vi "EminemNetworking.vi"(8 "error in (no error)":errorcluster) -> (0 "error out":errorcluster)   [LabVIEW 2023]
uses:
  EminemGlobals.vi
  <vilib>/Rock Robotics/Network Tables/NT Write Boolean.vi
  <vilib>/Rock Robotics/Network Tables/NT Write Number.vi
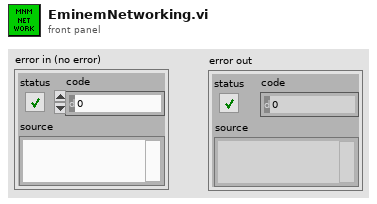
[diagram p1: front panel]
types:
  T1 = typedef "EminemStatesEnum.ctl" = enum16{"0-Init", "1-WaitForCmd", "2-Cancel", "3-ShootStart", "4-ShootRev", "5-RevUpStart", "6-ShootStartFeed&Timer", "7-ShootTimerOrSensorDone", "8-ShootDone", "9-AmpStart", "10-AmpUpToSpd?", "11-AmpStartFeed&Timer", "12-AmpTimerOrSensorDone", "13-AmpDone", "14-RevUpGetCmd"}
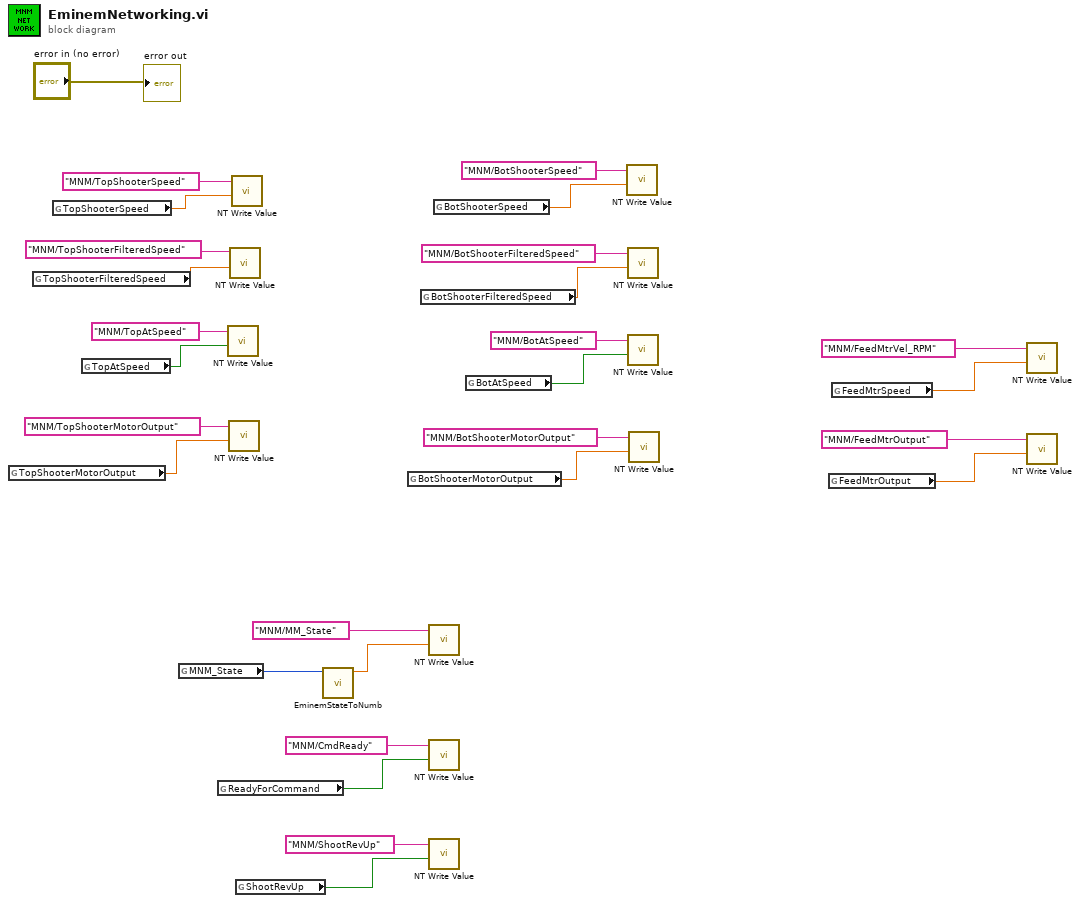
[diagram p0: block diagram]
diagram:
  n1 = global read "EminemGlobals.vi" "TopShooterMotorOutput"() -> (w12:dbl)
  n2 = global read "EminemGlobals.vi" "TopShooterFilteredSpeed"() -> (w18:dbl)
  n3 = global read "EminemGlobals.vi" "TopShooterSpeed"() -> (w17:dbl)
  n4 = global read "EminemGlobals.vi" "TopAtSpeed"() -> (w16:bool)
  n5 = global read "EminemGlobals.vi" "MNM_State"() -> (w7:T1)
  n6 = global read "EminemGlobals.vi" "ReadyForCommand"() -> (w10:bool)
  n7 = call-poly <vilib>:"NT Write Value.vi"("value"=w16, "name"="MNM/TopAtSpeed") -> ()  [unwired: 9 in, 1 out]
  n8 = call-poly <vilib>:"NT Write Value.vi"("value"=w12, "name"="MNM/TopShooterMotorOutput") -> ()  [unwired: 9 in, 1 out]
  n9 = call-poly <vilib>:"NT Write Value.vi"("value"=w18, "name"="MNM/TopShooterFilteredSpeed") -> ()  [unwired: 9 in, 1 out]
  n10 = call-poly <vilib>:"NT Write Value.vi"("value"=w17, "name"="MNM/TopShooterSpeed") -> ()  [unwired: 9 in, 1 out]
  n11 = global read "EminemGlobals.vi" "ShootRevUp"() -> (w1:bool)
  n12 = call "EminemStateToNumb.vi"("Eminim_state"=w7) -> ("StateNumber"=w5:dbl)  [unwired: 10 in]
  n13 = global read "EminemGlobals.vi" "BotShooterMotorOutput"() -> (w11:dbl)
  n14 = global read "EminemGlobals.vi" "BotShooterFilteredSpeed"() -> (w14:dbl)
  n15 = call-poly <vilib>:"NT Write Value.vi"("value"=w5, "name"="MNM/MM_State") -> ()  [unwired: 9 in, 1 out]
  n16 = call-poly <vilib>:"NT Write Value.vi"("value"=w10, "name"="MNM/CmdReady") -> ()  [unwired: 9 in, 1 out]
  n17 = call-poly <vilib>:"NT Write Value.vi"("value"=w1, "name"="MNM/ShootRevUp") -> ()  [unwired: 9 in, 1 out]
  n18 = global read "EminemGlobals.vi" "BotShooterSpeed"() -> (w15:dbl)
  n19 = global read "EminemGlobals.vi" "BotAtSpeed"() -> (w13:bool)
  n20 = call-poly <vilib>:"NT Write Value.vi"("value"=w15, "name"="MNM/BotShooterSpeed") -> ()  [unwired: 9 in, 1 out]
  n21 = call-poly <vilib>:"NT Write Value.vi"("value"=w14, "name"="MNM/BotShooterFilteredSpeed") -> ()  [unwired: 9 in, 1 out]
  n22 = call-poly <vilib>:"NT Write Value.vi"("value"=w13, "name"="MNM/BotAtSpeed") -> ()  [unwired: 9 in, 1 out]
  n23 = call-poly <vilib>:"NT Write Value.vi"("value"=w11, "name"="MNM/BotShooterMotorOutput") -> ()  [unwired: 9 in, 1 out]
  n24 = global read "EminemGlobals.vi" "FeedMtrOutput"() -> (w8:dbl)
  n25 = global read "EminemGlobals.vi" "FeedMtrSpeed"() -> (w3:dbl)
  n26 = call-poly <vilib>:"NT Write Value.vi"("value"=w3, "name"="MNM/FeedMtrVel_RPM") -> ()  [unwired: 9 in, 1 out]
  n27 = call-poly <vilib>:"NT Write Value.vi"("value"=w8, "name"="MNM/FeedMtrOutput") -> ()  [unwired: 9 in, 1 out]
  "error out" <- "error in (no error)"
